vi "Main.vi"() -> ()   [LabVIEW 2013]
uses:
  Ch1.ctl
panel:
  in  "Крутити вліво n разів":bool
  in  "Крутити вліво безкічечно":bool
  out "2D Picture":picture
  in  "Затримка, с":i32
  in  "Exit":bool
  in  "n =":i32
  in  "Крутити вправо n разів":bool
  in  "Крутити вправо безкічечно":bool
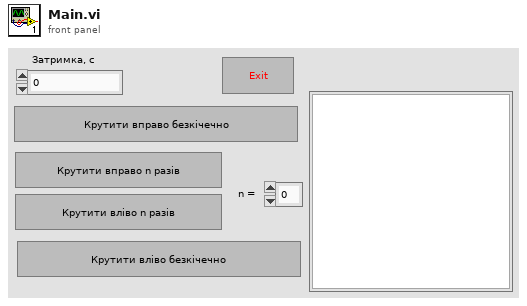
[diagram p1: front panel]
types:
  T1 = typedef "Ch1.ctl" = enum16{"def", "1 Start", "1 Start n", "2 Start", "2 Start n", "Exit", "Stop"}
  T2 = typedef "imagedata.ctl" = cluster{"image type":i32, "image depth":i32, "image":u8[], "mask":u8[], "colors":u32[], "Rectangle":cluster{"left":i16, "top":i16, "right":i16, "bottom":i16}}
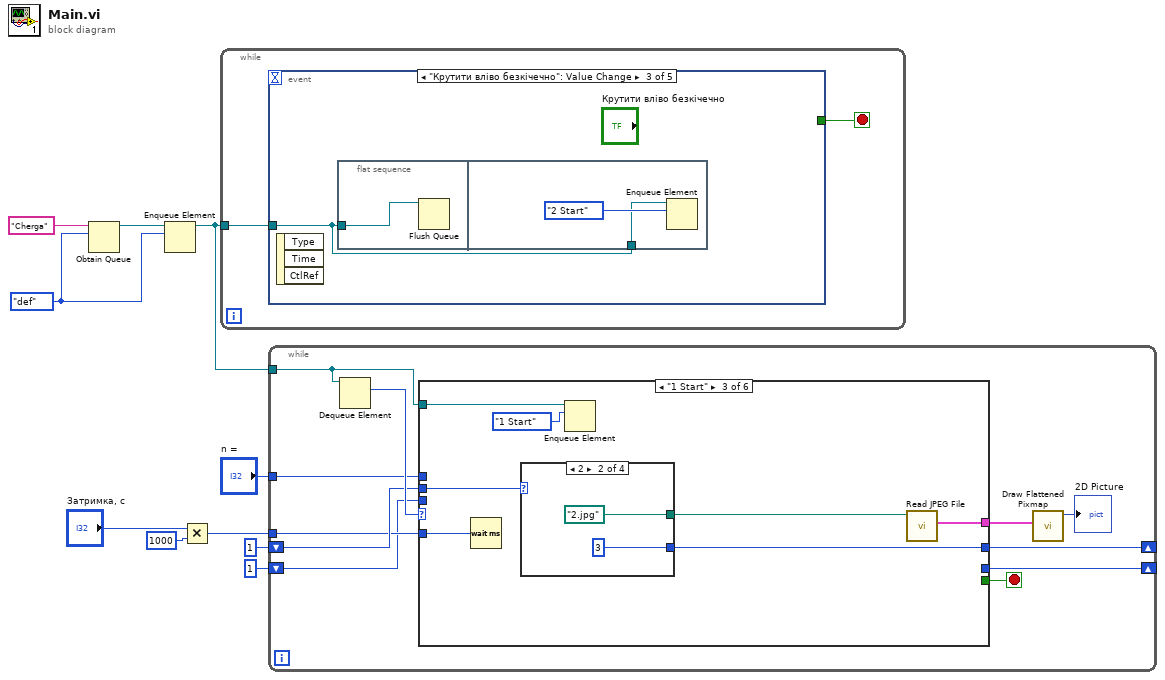
[diagram p0: block diagram]
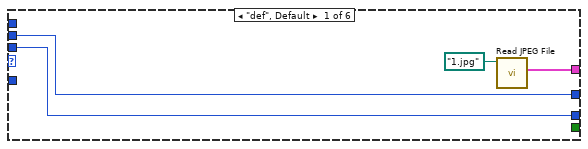
[diagram p2: hidden frame]
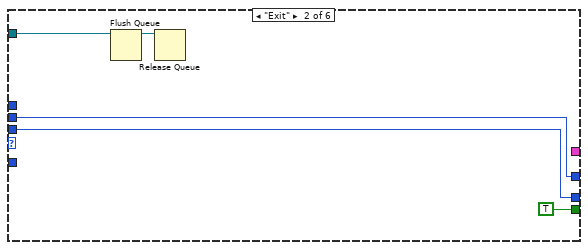
[diagram p3: hidden frame]
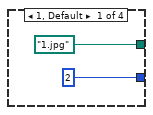
[diagram p4: hidden frame]
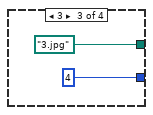
[diagram p5: hidden frame]
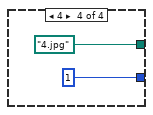
[diagram p6: hidden frame]
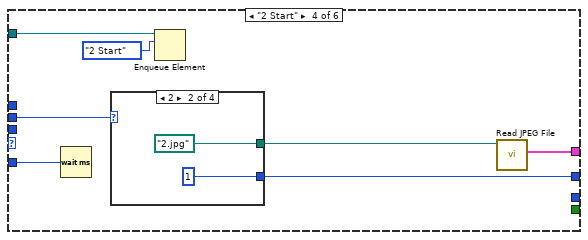
[diagram p7: hidden frame]
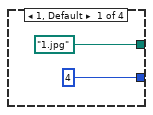
[diagram p8: hidden frame]
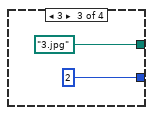
[diagram p9: hidden frame]
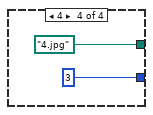
[diagram p10: hidden frame]
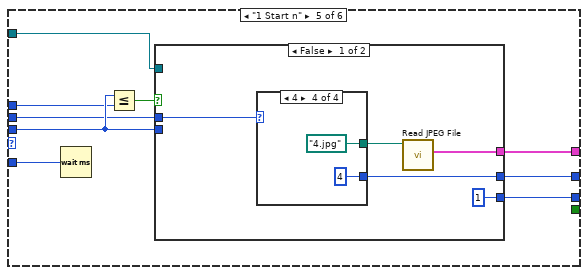
[diagram p11: hidden frame]
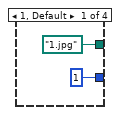
[diagram p12: hidden frame]
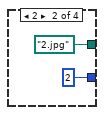
[diagram p13: hidden frame]
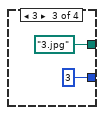
[diagram p14: hidden frame]
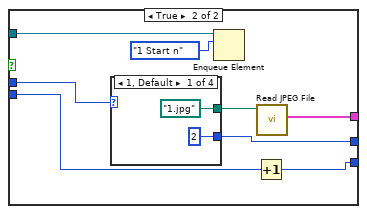
[diagram p15: hidden frame]
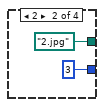
[diagram p16: hidden frame]
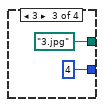
[diagram p17: hidden frame]
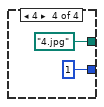
[diagram p18: hidden frame]
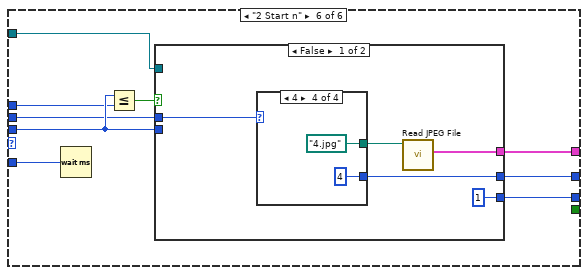
[diagram p19: hidden frame]
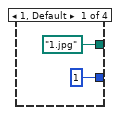
[diagram p20: hidden frame]
diagram:
  w8 = Ch1."def" ("Enum")
  n1 = Obtain Queue(name (unnamed)="Cherga", element data type=w8) -> (queue out=w9:refnum<queue>)  [unwired: 3 in, 2 out]
  n2 = Enqueue Element(queue=w9, element=w8) -> (queue out=w7:refnum<queue>)  [unwired: 2 in, 2 out]
  n3 = Multiply(x="Затримка, с", y=1000) -> (x*y=w3:i32)
  n4 = while {
    tunnel: w7 -> [w12]
    stop <- w11 stop-if-true
    n5 = event shown="[2] \"Крутити вліво безкічечно\": Value Change" {
      selector: _ -> [_ _ _ _ _]
      dyn-events: _ -> [_ _ _ _ _]
      timeout: _ -> [_ _ _ _ _]
      tunnel: w12 -> [w15 w16 w20 w24 w28]
      tunnel: [TRUE _ _ _ _] -> w11
      event "Exit": Value Change {
        n6 = event-data() -> ()  [unwired: 1 in, 3 out]
        n7 = Enqueue Element At Opposite End(queue=w15, element=Ch1."Exit" ("Enum")) -> ()  [unwired: 2 in, 3 out]
      }
      event "Крутити вправо безкічечно": Value Change {
        n8 = event-data() -> ()  [unwired: 1 in, 3 out]
        n9 = flat-sequence {
          tunnel: w16 -> [w17]
          tunnel: w16 -> [w18]
          frame #0 {
            n10 = Flush Queue(queue=w17) -> ()  [unwired: 1 in, 3 out]
          }
          frame #1 {
            n11 = Enqueue Element(queue=w18, element=Ch1."1 Start" ("Enum")) -> ()  [unwired: 2 in, 3 out]
          }
        }
      }
      event "Крутити вліво безкічечно": Value Change {
        n12 = event-data() -> ()  [unwired: 1 in, 3 out]
        n13 = flat-sequence {
          tunnel: w20 -> [w21]
          tunnel: w20 -> [w22]
          frame #0 {
            n14 = Flush Queue(queue=w21) -> ()  [unwired: 1 in, 3 out]
          }
          frame #1 {
            n15 = Enqueue Element(queue=w22, element=Ch1."2 Start" ("Enum")) -> ()  [unwired: 2 in, 3 out]
          }
        }
      }
      event "Крутити вправо n разів": Value Change {
        n16 = event-data() -> ()  [unwired: 1 in, 3 out]
        n17 = flat-sequence {
          tunnel: w24 -> [w25]
          tunnel: w24 -> [w26]
          frame #0 {
            n18 = Flush Queue(queue=w25) -> ()  [unwired: 1 in, 3 out]
          }
          frame #1 {
            n19 = Enqueue Element(queue=w26, element=Ch1."1 Start n" ("Enum")) -> ()  [unwired: 2 in, 3 out]
          }
        }
      }
      event "Крутити вліво n разів": Value Change {
        n20 = event-data() -> ()  [unwired: 1 in, 3 out]
        n21 = flat-sequence {
          tunnel: w28 -> [w29]
          tunnel: w28 -> [w30]
          frame #0 {
            n22 = Flush Queue(queue=w29) -> ()  [unwired: 1 in, 3 out]
          }
          frame #1 {
            n23 = Enqueue Element(queue=w30, element=Ch1."2 Start n" ("Enum")) -> ()  [unwired: 2 in, 3 out]
          }
        }
      }
    }
  }
  n24 = while {
    tunnel: w7 -> [w41]
    shift-right: [w33] -> _
    shift-left: 1 -> [w40]
    tunnel: w3 -> [w38]
    shift-right: [w34] -> _
    shift-left: 1 -> [w35]
    tunnel: "n =" -> [w32]
    stop <- w39 stop-if-true
    n25 = Dequeue Element(queue=w41) -> (element=w42:T1)  [unwired: 2 in, 3 out]
    n26 = case shown="\"1 Start\"" w42 {
      tunnel: w41 -> [_ w51 w57 w72 w87 w125]
      tunnel: w40 -> [w46 w48 w55 w70 w85 w123]
      tunnel: [w45 w47 _ _ w89 w127] -> w34
      tunnel: [_ TRUE _ _ _ _] -> w39
      tunnel: w38 -> [_ _ w56 w71 w88 w126]
      tunnel: [w43 _ w53 w68 w83 w121] -> w36
      tunnel: w35 -> [w45 w47 _ _ w86 w124]
      tunnel: [w46 w48 w52 w67 w84 w122] -> w33
      tunnel: w32 -> [_ _ _ _ w82 w120]
      frame "def", Default {
        n27 = call <vilib>:"Read JPEG File.vi"("path to JPEG file"=path "1.jpg") -> ("image data"=w43:T2)  [unwired: 8 in, 2 out]
      }
      frame "Exit" {
        n28 = Flush Queue(queue=w51) -> (queue out=w50:refnum<queue>)  [unwired: 1 in, 2 out]
        n29 = Release Queue(queue=w50) -> ()  [unwired: 2 in, 3 out]
      }
      frame "1 Start" {
        n30 = Wait (ms)(milliseconds to wait=w56) -> ()  [unwired: 1 out]
        n31 = case shown="2" w55 {
          tunnel: [path "1.jpg" path "2.jpg" path "3.jpg" path "4.jpg"] -> w54
          tunnel: [2 3 4 1] -> w52
          frame 1, Default {
          }
          frame 2 {
          }
          frame 3 {
          }
          frame 4 {
          }
        }
        n32 = Enqueue Element(queue=w57, element=Ch1."1 Start" ("Enum")) -> ()  [unwired: 2 in, 3 out]
        n33 = call <vilib>:"Read JPEG File.vi"("path to JPEG file"=w54) -> ("image data"=w53:T2)  [unwired: 8 in, 2 out]
      }
      frame "2 Start" {
        n34 = Wait (ms)(milliseconds to wait=w71) -> ()  [unwired: 1 out]
        n35 = case shown="2" w70 {
          tunnel: [path "1.jpg" path "2.jpg" path "3.jpg" path "4.jpg"] -> w69
          tunnel: [4 1 2 3] -> w67
          frame 1, Default {
          }
          frame 2 {
          }
          frame 3 {
          }
          frame 4 {
          }
        }
        n36 = Enqueue Element(queue=w72, element=Ch1."2 Start" ("Enum")) -> ()  [unwired: 2 in, 3 out]
        n37 = call <vilib>:"Read JPEG File.vi"("path to JPEG file"=w69) -> ("image data"=w68:T2)  [unwired: 8 in, 2 out]
      }
      frame "1 Start n" {
        n38 = Wait (ms)(milliseconds to wait=w88) -> ()  [unwired: 1 out]
        n39 = Less Or Equal?(x=w86, y=w82) -> (x <= y?=w90:bool)
        n40 = case shown="False" w90 {
          tunnel: w86 -> [_ w111]
          tunnel: [1 w110] -> w89
          tunnel: w87 -> [_ w108]
          tunnel: w85 -> [w92 w106]
          tunnel: [w93 w105] -> w84
          tunnel: [w94 w104] -> w83
          frame False {
            n41 = case shown="4" w92 {
              tunnel: [path "1.jpg" path "2.jpg" path "3.jpg" path "4.jpg"] -> w95
              tunnel: [1 2 3 4] -> w93
              frame 1, Default {
              }
              frame 2 {
              }
              frame 3 {
              }
              frame 4 {
              }
            }
            n42 = call <vilib>:"Read JPEG File.vi"("path to JPEG file"=w95) -> ("image data"=w94:T2)  [unwired: 8 in, 2 out]
          }
          frame True {
            n43 = case shown="1, Default" w106 {
              tunnel: [path "1.jpg" path "2.jpg" path "3.jpg" path "4.jpg"] -> w107
              tunnel: [2 3 4 1] -> w105
              frame 1, Default {
              }
              frame 2 {
              }
              frame 3 {
              }
              frame 4 {
              }
            }
            n44 = Enqueue Element(queue=w108, element=Ch1."1 Start n" ("Enum")) -> ()  [unwired: 2 in, 3 out]
            n45 = Increment(x=w111) -> (x+1=w110:i32)
            n46 = call <vilib>:"Read JPEG File.vi"("path to JPEG file"=w107) -> ("image data"=w104:T2)  [unwired: 8 in, 2 out]
          }
        }
      }
      frame "2 Start n" {
        n47 = Wait (ms)(milliseconds to wait=w126) -> ()  [unwired: 1 out]
        n48 = Less Or Equal?(x=w124, y=w120) -> (x <= y?=w128:bool)
        n49 = case shown="False" w128 {
          tunnel: w124 -> [_ w149]
          tunnel: [1 w148] -> w127
          tunnel: w125 -> [_ w146]
          tunnel: w123 -> [w130 w144]
          tunnel: [w131 w143] -> w122
          tunnel: [w132 w142] -> w121
          frame False {
            n50 = case shown="4" w130 {
              tunnel: [path "1.jpg" path "2.jpg" path "3.jpg" path "4.jpg"] -> w133
              tunnel: [1 2 3 4] -> w131
              frame 1, Default {
              }
              frame 2 {
              }
              frame 3 {
              }
              frame 4 {
              }
            }
            n51 = call <vilib>:"Read JPEG File.vi"("path to JPEG file"=w133) -> ("image data"=w132:T2)  [unwired: 8 in, 2 out]
          }
          frame True {
            n52 = case shown="4" w144 {
              tunnel: [path "1.jpg" path "2.jpg" path "3.jpg" path "4.jpg"] -> w145
              tunnel: [4 1 2 3] -> w143
              frame 1, Default {
              }
              frame 2 {
              }
              frame 3 {
              }
              frame 4 {
              }
            }
            n53 = Enqueue Element(queue=w146, element=Ch1."2 Start n" ("Enum")) -> ()  [unwired: 2 in, 3 out]
            n54 = Increment(x=w149) -> (x+1=w148:i32)
            n55 = call <vilib>:"Read JPEG File.vi"("path to JPEG file"=w145) -> ("image data"=w142:T2)  [unwired: 8 in, 2 out]
          }
        }
      }
    }
    n56 = call <vilib>:"Draw Flattened Pixmap.vi"("image data"=w36) -> ("new picture"=→"2D Picture":picture)  [unwired: 8 in]
  }
